vi "Username Password (SubVI).vi"(1 "Username":string, 2 "Password":string) -> (0 "0, 1":i16)   [LabVIEW 2020]
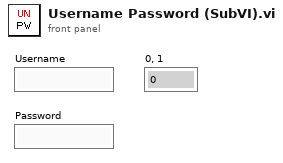
[diagram p1: front panel]
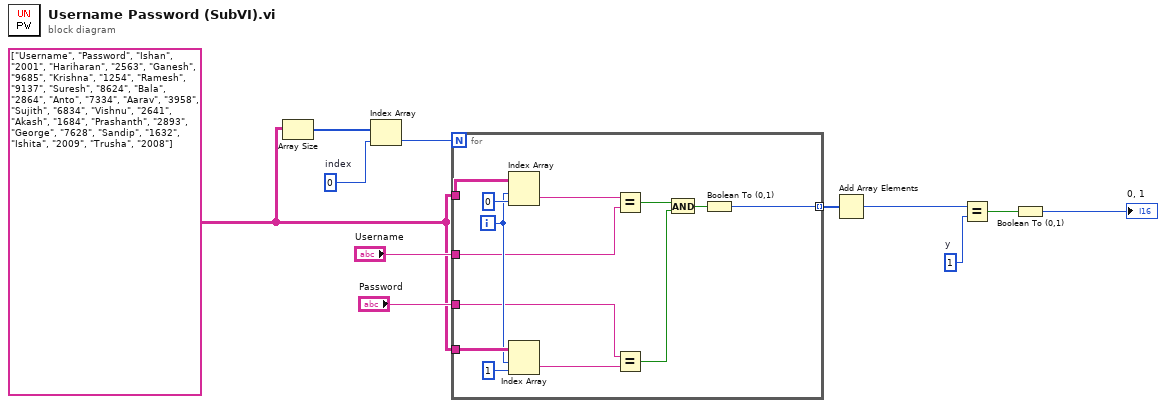
[diagram p0: block diagram]
diagram:
  w4 = string[][] [["Username", "Password"], ["Ishan", "2001"], ["Hariharan", "2563"], ["Ganesh", "9685"], ["Krishna", "1254"], ["Ramesh", "9137"], ["Suresh", "8624"], ["Bala", "2864"], ["Anto", "7334"], ["Aarav", "3958"], ["Sujith", "6834"], ["Vishnu", "2641"], ["Akash", "1684"], ["Prashanth", "2893"], ["George", "7628"], ["Sandip", "1632"], ["Ishita", "2009"], ["Trusha", "2008"]] ("Array")
  w7 = i16 1  # y
  w2 = 0  # index
  n1 = Array Size(array=w4) -> (size(s)=w1:i32[])
  n2 = Index Array "Index Array"(array=w1, index=w2) -> (element=w3:i32)
  n3 = for {
    N: w3 -> [_]
    tunnel: w4 -> [w24]
    tunnel: w4 -> [w22]
    tunnel: [w15] -> w5 mode=indexing
    tunnel: "Username" -> [w13]
    tunnel: "Password" -> [w12]
    i -> [w20]
    n4 = Index Array "Index Array"(array=w24, index (row)=w20, index (col)=0 ("disabled index (col)")) -> (element=w19:string)
    n5 = Index Array "Index Array"(array=w22, index (row)=w20, index (col)=1 ("disabled index (col)")) -> (element=w18:string)
    n6 = Equal?(x=w19, y=w13) -> (x = y?=w17:bool)
    n7 = Equal?(x=w12, y=w18) -> (x = y?=w16:bool)
    n8 = And(x=w17, y=w16) -> (x .and. y?=w14:bool)
    n9 = Boolean To (0,1)(Boolean=w14) -> (0, 1=w15:i16)
  }
  n10 = Add Array Elements(numeric array=w5) -> (sum=w6:i16)
  n11 = Equal?(x=w6, y=w7) -> (x = y?=w8:bool)
  n12 = Boolean To (0,1)(Boolean=w8) -> (0, 1=→"0, 1":i16)
